vi "Create Sort Keys.vi"(8 "error in (no error)":errorcluster, 11 "Repeatability Results":T1[](array[typedef]) {"Repeatability Percent FS" format="%#_3g"}) -> (0 "error out":errorcluster, 3 "Sort Keys":dbl[](array[numeric]))   [LabVIEW 2026, in "Analysis.lvlib"]
uses:
  Analysis.lvlib
  Repeatability Result.ctl
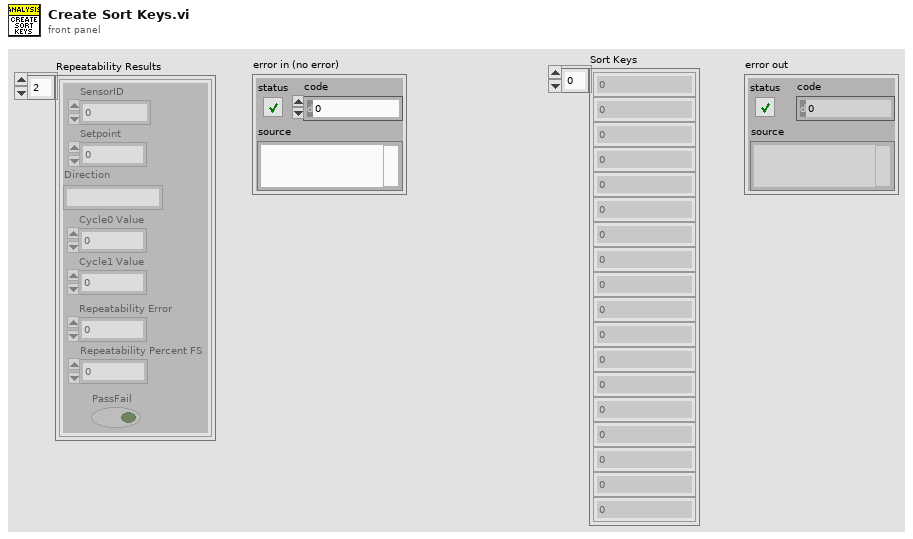
[diagram p1: front panel]
types:
  T1 = typedef "Analysis.lvlib/Repeatability Result.ctl" = cluster{"Setpoint":dbl, "Cycle0 Value":dbl, "SensorID":i32, "Cycle1 Value":dbl, "Repeatability Error":dbl, "Direction":string, "Repeatability Percent FS":dbl, "PassFail":bool}
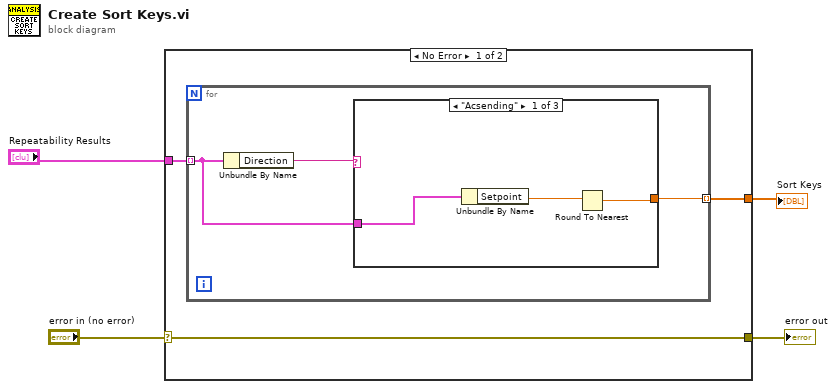
[diagram p0: block diagram]
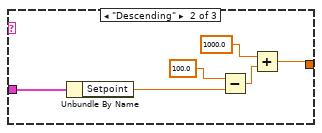
[diagram p2: hidden frame]
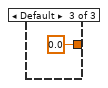
[diagram p3: hidden frame]
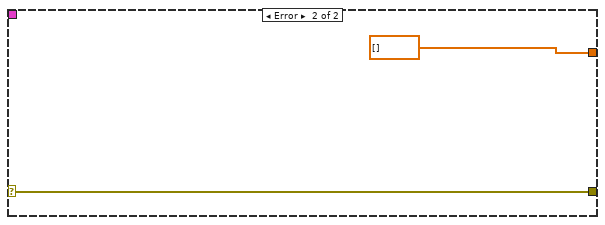
[diagram p4: hidden frame]
diagram:
  n1 = case shown="No Error" "error in (no error)" {
    selector: "error in (no error)" -> [w6 w22]
    tunnel: "Repeatability Results" -> [w7 _]
    tunnel: [w6 w22] -> w3
    tunnel: [w5 dbl[] []] -> w2
    frame No Error {
      n2 = for {
        tunnel: w7 -> [w9] mode=indexing
        tunnel: [w8] -> w5 mode=indexing
        n3 = Unbundle By Name(w9) -> ("Direction"=w10:string)
        n4 = case shown="\"Acsending\"" w10 {
          tunnel: w9 -> [w13 w19 _]
          tunnel: [w11 w14 0.0 ("Setpoint")] -> w8
          frame "Acsending" {
            n5 = Unbundle By Name(w13) -> ("Setpoint"=w12:dbl)
            n6 = Round To Nearest(number=w12) -> (nearest integer value=w11:dbl)
          }
          frame "Descending" {
            n7 = Unbundle By Name(w19) -> ("Setpoint"=w17:dbl)
            n8 = Subtract(x=100.0, y=w17) -> (x-y=w16:dbl)
            n9 = Add(x=1000.0, y=w16) -> (x+y=w14:dbl)
          }
          frame Default {
          }
        }
      }
    }
    frame Error {
    }
  }
  "Sort Keys" <- w2
  "error out" <- w3
